vi "Lookup Pref Value.vi"(8 "error in (no error)":errorcluster, 10 "Pref Hierarchy":string[](array[string]), 11 "Pref Group in":refnum<class "Pref Group.lvclass">) -> (0 "error out":errorcluster, 2 "Value":string, 3 "Pref Group out":refnum<class "Pref Group.lvclass">)   [LabVIEW 2020, in "User Prefs.lvlib" / "Pref Group.lvclass"]
uses:
  Pref Group.lvclass
  Pref Group.lvclass/Pref Group.ctl
  lv-cdm/CDM-Config/Config Manager/Config Manager.lvclass
  lv-cdm/CDM-Config/Config Element/Config Element.lvclass
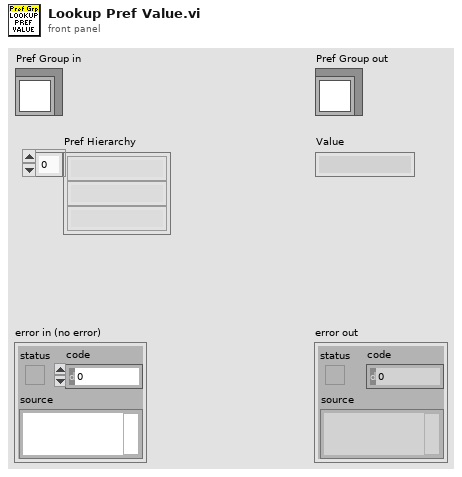
[diagram p1: front panel]
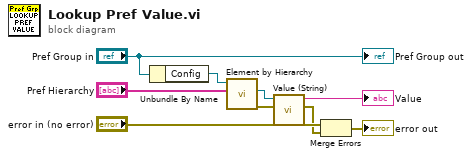
[diagram p0: block diagram]
diagram:
  n1 = Unbundle By Name("Pref Group in") -> ("Config"=w7:refnum<class "Config Manager.lvclass">)
  n2 = call "Element by Hierarchy.vi"("Hierarchy"="Pref Hierarchy", "Config Manager in"=w7) -> ("error out"=w4:errorcluster, "Config Element"=w5:refnum<class "Config Element.lvclass">)  [unwired: 7 in, 1 out]
  n3 = call "Value (String).vi"("error in (no error)"=w4, "Config Element in"=w5) -> ("error out"=w1:errorcluster, "String Value"=→"Value":string)  [unwired: 8 in]
  n4 = Merge Errors("error in (no error)", w1) -> (→"error out":errorcluster)
  "Pref Group out" <- "Pref Group in"
